vi "FGV_VISA_Comm.vi"(7 "Write?":bool, 8 "error in":errorcluster caption="错误输入", 10 "Host VISA resource name":refnum<visa-resource-name>="COM4", 11 "ACC VISA resource name":refnum<visa-resource-name>="COM4") -> (0 "error out":errorcluster caption="错误输出", 1 "Host VISA resource name out":refnum<visa-resource-name>="COM4", 2 "ACC Interface Information":string, 3 "ACC VISA resource name out":refnum<visa-resource-name>="COM4", 4 "Host Interface Information":string)   [LabVIEW 2020]
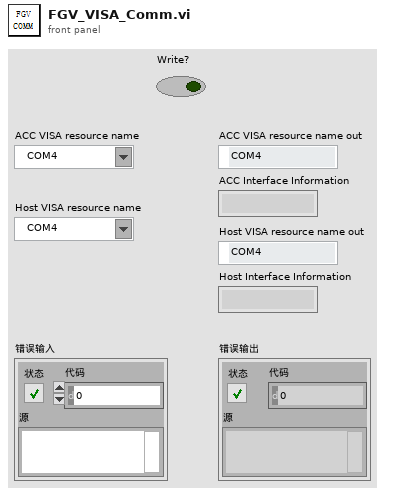
[diagram p1: front panel]
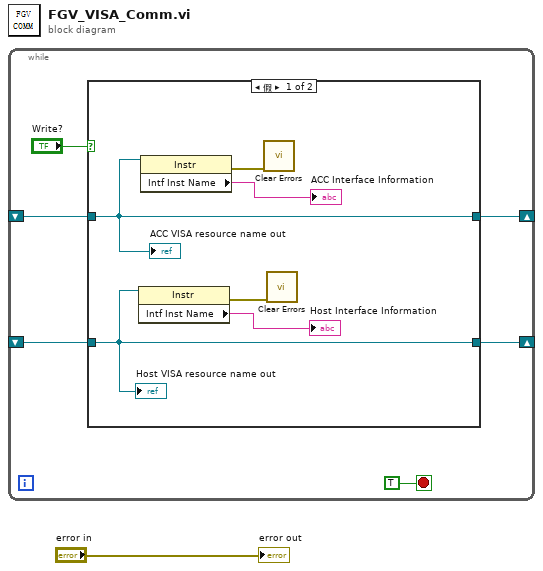
[diagram p0: block diagram]
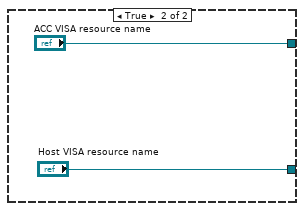
[diagram p2: hidden frame]
diagram:
  n1 = while {
    shift-right: [w5] -> _
    shift-left: _ -> [w4]
    shift-right: [w3] -> _
    shift-left: _ -> [w2]
    stop <- TRUE stop-if-true
    n2 = case shown="假" "Write?" {
      tunnel: [w13 "ACC VISA resource name"] -> w5
      tunnel: w4 -> [w13 _]
      tunnel: [w10 "Host VISA resource name"] -> w3
      tunnel: w2 -> [w10 _]
      frame False {
        n3 = property class="Instr"(reference=w10) -> (error out=w8:errorcluster, "Intf Inst Name"=→"Host Interface Information":string)  [unwired: 1 in, 1 out]
        n4 = property class="Instr"(reference=w13) -> (error out=w11:errorcluster, "Intf Inst Name"=→"ACC Interface Information":string)  [unwired: 1 in, 1 out]
        n5 = call <vilib>:"Clear Errors.vi"("error in (no error)"=w11) -> ()  [unwired: 5 in, 2 out]
        n6 = call <vilib>:"Clear Errors.vi"("error in (no error)"=w8) -> ()  [unwired: 5 in, 2 out]
        "ACC VISA resource name out" <- w13
        "Host VISA resource name out" <- w10
      }
      frame True {
      }
    }
  }
  "error out" <- "error in"
